vi "pulse_generator_data.vi"(3 "PG Data":refnum<vi>, 4 "Record dP Data":refnum<vi>, 5 "queue in":refnum<queue>, 6 "Stop! Refnum":refnum<vi>, 7 "Recording Progressbar":refnum<vi>, 8 "Seesion Start Time":timestamp, 9 "Pulse Generator Chart Refnums":T3, 10 "Pulse Generator Offsets and Data Saving Controls Refnums":T2, 11 "Pulse Generator Measurement Refnums":T1) -> ()   [LabVIEW 2017]
uses:
  pulse_generator_data_charts_refnums.ctl
  pulse_generator_data_controls_refnums.ctl
  pulse_generator_data_refnums.ctl
  <vilib>/Waveform/WDTOps.llb/WDT Get Waveform Time Array DBL.vi
panel:
  out "size(s)":i32[](graph)
  out "Sampling Rate":refnum<vi>
  out "Recording Duration":refnum<vi>
  out "Camera Voltage Chart":refnum<vi>
  out "Abs Tank Pressure Chart":refnum<vi>
  out "Pitot dP Chart":refnum<vi>
  out "Pulse Generator to Test Section dP Chart":refnum<vi>
  out "W1-7 dP":refnum<vi>
  out "W1-4 dP":refnum<vi>
  out "Mass Flow Rate":refnum<vi>
  out "Liquid Sat Pressure":refnum<vi>
  out "Liquid Temperature":refnum<vi>
  out "Vapor Sat Pressure":refnum<vi>
  out "Vapor Temperature":refnum<vi>
  out "Pitot dP":refnum<vi>
  out "PG to TS dP":refnum<vi>
  out "Pitot Current":refnum<vi>
  out "PG Abs Pressure":refnum<vi>
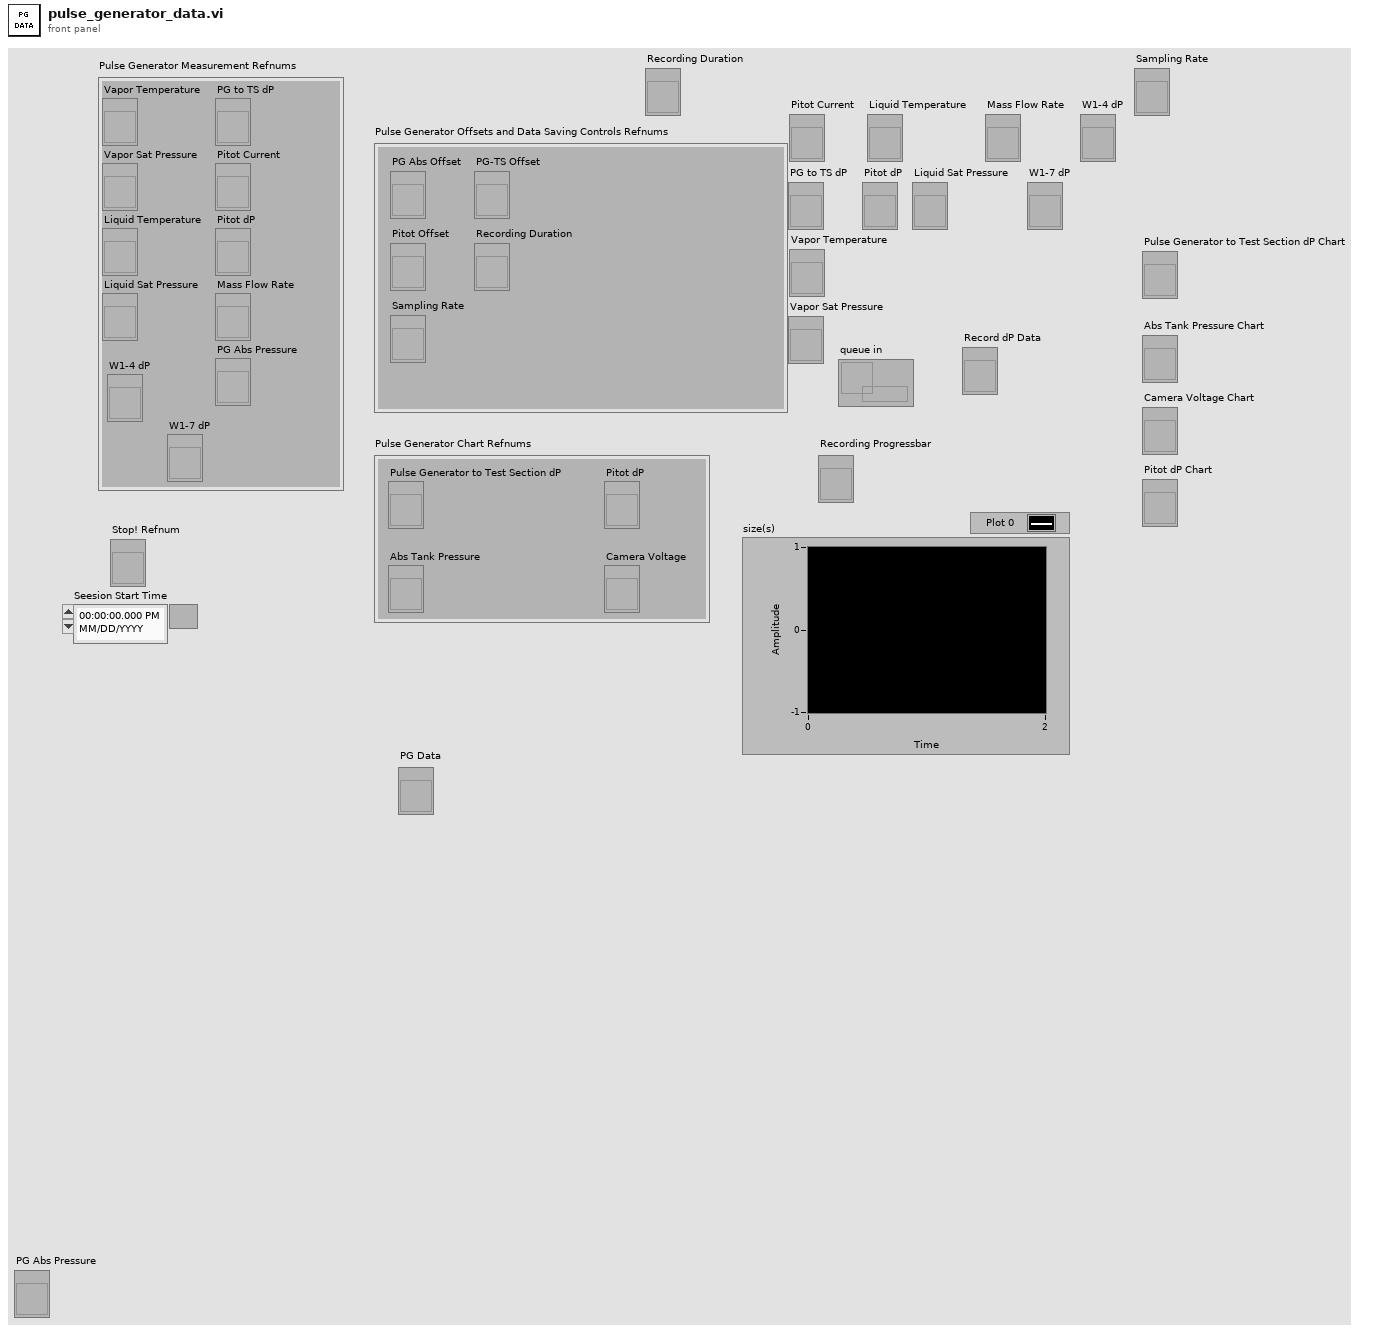
[diagram p1: front panel]
types:
  T1 = typedef "pulse_generator_data_refnums.ctl" = cluster{"Vapor Temperature":refnum<vi>, "Vapor Sat Pressure":refnum<vi>, "Liquid Temperature":refnum<vi>, "Liquid Sat Pressure":refnum<vi>, "PG to TS dP":refnum<vi>, "Pitot Current":refnum<vi>, "Pitot dP":refnum<vi>, "Mass Flow Rate":refnum<vi>, "PG Abs Pressure":refnum<vi>, "W1-4 dP":refnum<vi>, "W1-7 dP":refnum<vi>}
  T2 = typedef "pulse_generator_data_controls_refnums.ctl" = cluster{"PG Abs Offset":refnum<vi>, "Pitot Offset":refnum<vi>, "PG-TS Offset":refnum<vi>, "Recording Duration":refnum<vi>, "Sampling Rate":refnum<vi>}
  T3 = typedef "pulse_generator_data_charts_refnums.ctl" = cluster{"Pulse Generator to Test Section dP":refnum<vi>, "Pitot dP":refnum<vi>, "Abs Tank Pressure":refnum<vi>, "Camera Voltage":refnum<vi>}
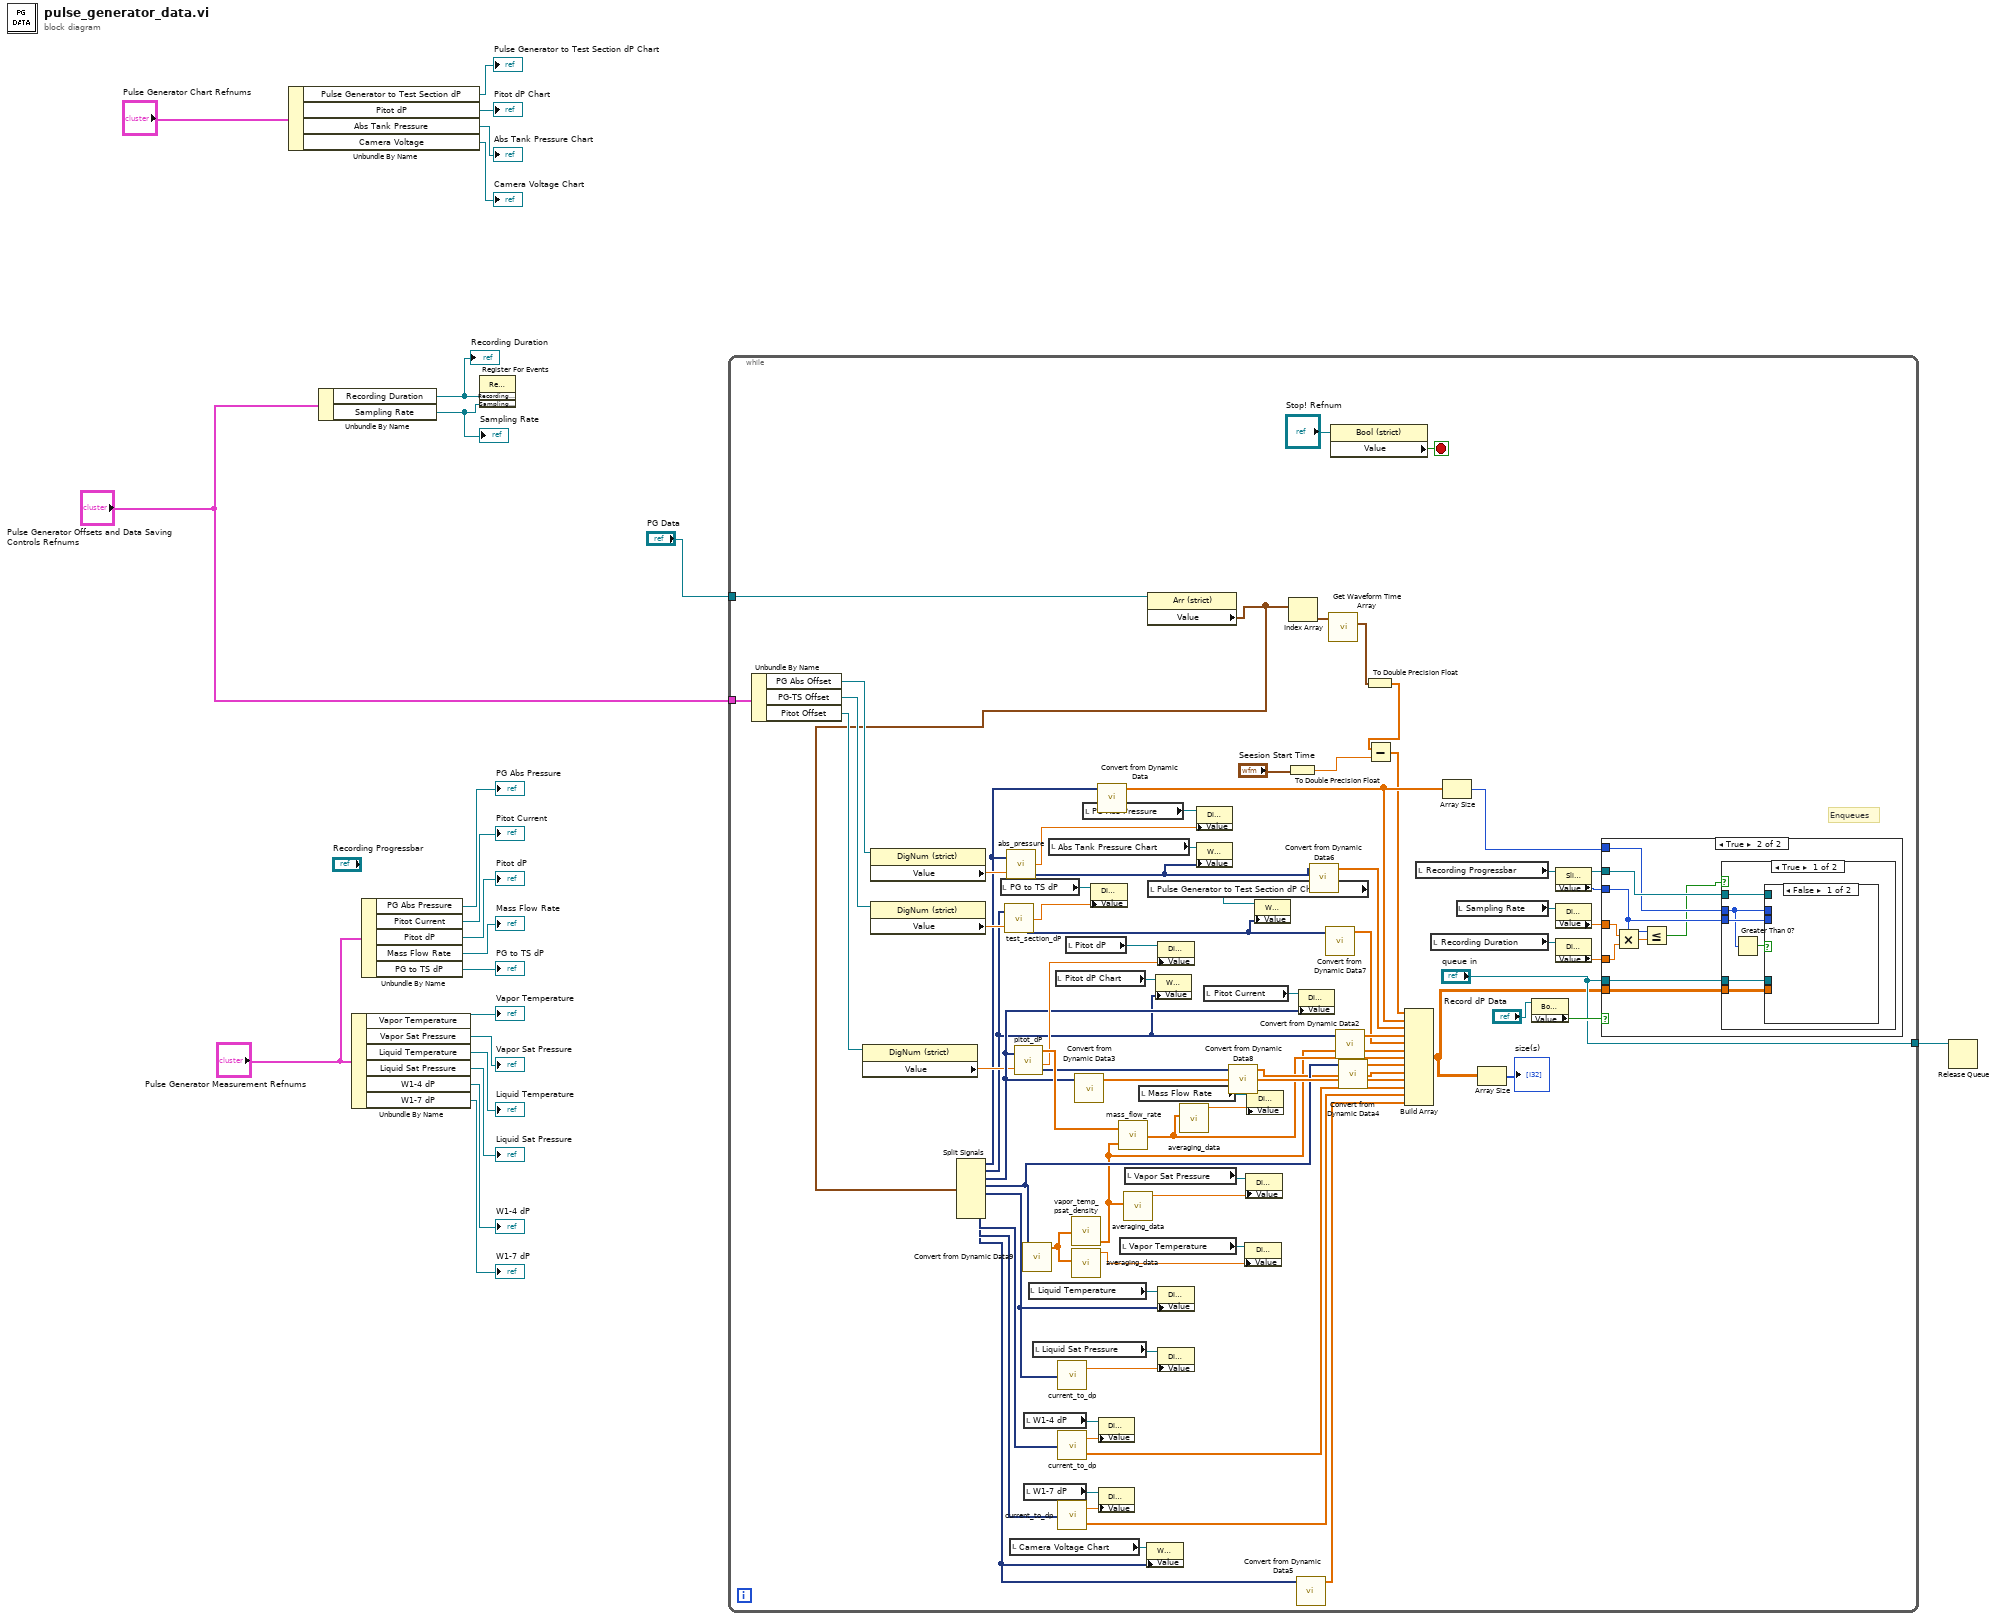
[diagram p0: block diagram]
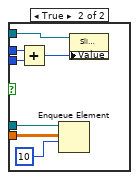
[diagram p3: hidden frame]
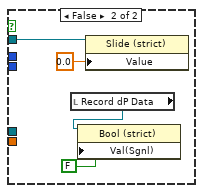
[diagram p4: hidden frame]
diagram:
  n1 = Unbundle By Name("Pulse Generator Chart Refnums") -> ("Pulse Generator to Test Section dP"=→"Pulse Generator to Test Section dP Chart":refnum<vi>, "Pitot dP"=→"Pitot dP Chart":refnum<vi>, "Abs Tank Pressure"=→"Abs Tank Pressure Chart":refnum<vi>, "Camera Voltage"=→"Camera Voltage Chart":refnum<vi>)
  n2 = Unbundle By Name("Pulse Generator Offsets and Data Saving Controls Refnums") -> ("Recording Duration"=w4:refnum<vi>, "Sampling Rate"=w3:refnum<vi>)
  "Recording Duration" <- w4
  "Sampling Rate" <- w3
  n3 = Unbundle By Name("Pulse Generator Measurement Refnums") -> ("Vapor Temperature"=→"Vapor Temperature":refnum<vi>, "Vapor Sat Pressure"=→"Vapor Sat Pressure":refnum<vi>, "Liquid Temperature"=→"Liquid Temperature":refnum<vi>, "Liquid Sat Pressure"=→"Liquid Sat Pressure":refnum<vi>, "W1-4 dP"=→"W1-4 dP":refnum<vi>, "W1-7 dP"=→"W1-7 dP":refnum<vi>)
  n4 = Unbundle By Name("Pulse Generator Measurement Refnums") -> ("PG Abs Pressure"=→"PG Abs Pressure":refnum<vi>, "Pitot Current"=→"Pitot Current":refnum<vi>, "Pitot dP"=→"Pitot dP":refnum<vi>, "Mass Flow Rate"=→"Mass Flow Rate":refnum<vi>, "PG to TS dP"=→"PG to TS dP":refnum<vi>)
  n5 = register-events(w4, w3) -> ()  [unwired: 2 in, 2 out]
  n6 = while {
    tunnel: "Pulse Generator Offsets and Data Saving Controls Refnums" -> [w99]
    tunnel: ["queue in"] -> w6
    tunnel: "PG Data" -> [w30]
    stop <- w100 stop-if-true
    # "Enqueues"
    n7 = Unbundle By Name(w99) -> ("PG Abs Offset"=w98:refnum<vi>, "PG-TS Offset"=w97:refnum<vi>, "Pitot Offset"=w96:refnum<vi>)
    n8 = property class="DigNum (strict)"(reference=w96) -> ("Value"=w48:dbl)  [unwired: 1 in, 2 out]
    n9 = property class="DigNum (strict)"(reference=w98) -> ("Value"=w95:dbl)  [unwired: 1 in, 2 out]
    n10 = property class="DigNum (strict)"(reference=w97) -> ("Value"=w52:dbl)  [unwired: 1 in, 2 out]
    n11 = local read "PG to TS dP"() -> (w94:refnum<vi>)
    n12 = local read "Camera Voltage Chart"() -> (w73:refnum<vi>)
    n13 = local read "W1-4 dP"() -> (w83:refnum<vi>)
    n14 = local read "W1-7 dP"() -> (w80:refnum<vi>)
    n15 = local read "Liquid Temperature"() -> (w87:refnum<vi>)
    n16 = local read "Liquid Sat Pressure"() -> (w89:refnum<vi>)
    n17 = local read "Abs Tank Pressure Chart"() -> (w76:refnum<vi>)
    n18 = local read "Pitot dP Chart"() -> (w75:refnum<vi>)
    n19 = local read "Pitot dP"() -> (w92:refnum<vi>)
    n20 = local read "PG Abs Pressure"() -> (w50:refnum<vi>)
    n21 = local read "Vapor Temperature"() -> (w85:refnum<vi>)
    n22 = local read "Vapor Sat Pressure"() -> (w78:refnum<vi>)
    n23 = local read "Mass Flow Rate"() -> (w90:refnum<vi>)
    n24 = property class="Arr (strict)"(reference=w30) -> ("Value"=w29:waveform(dbl)[])  [unwired: 1 in, 2 out]
    n25 = Split Signals(w29) -> (w37:dynamicdata, w46:dynamicdata, w55:dynamicdata, w53:dynamicdata, w86:dynamicdata, w82:dynamicdata, w81:dynamicdata, w64:dynamicdata)  [unwired: 8 in]
    n26 = call "test_section_dP.vi"("dP Voltage"=w46, "Offset[Pa]"=w52) -> ("Adj dP"=w71:dbl, "Adj dP Array"=w40:dynamicdata)  [unwired: 1 out]
    n27 = call "abs_pressure.vi"("Input Voltage"=w37, "Offset[Pa]"=w95) -> ("Adj Absolute Pressure"=w72:dbl, "Adj Absolute Pressure Array"=w42:dynamicdata)  [unwired: 1 out]
    n28 = call "pitot_dP.vi"("Pitot Current"=w55, "Pitot Offset [Pa]"=w48) -> ("dP H2O"=w91:dbl[], "Adj dP [Pa]"=w74:dbl, "Adj dP [Pa] Array"=w38:dynamicdata)  [unwired: 1 out]
    n29 = call "Convert from Dynamic Data9"("Dynamic Data Type"=w53) -> ("Array"=w26:dbl[])  [unwired: 3 in]
    n30 = call "current_to_dp.vi"("Current [A]"=w86) -> ("dP [Pa]"=w88:dbl)  [unwired: 1 out]
    n31 = call "current_to_dp.vi"("Current [A]"=w82) -> ("dP [Pa]"=w84:dbl, "dP Array [Pa]"=w70:dbl[])
    n32 = call "current_to_dp.vi"("Current [A]"=w81) -> ("dP [Pa]"=w79:dbl, "dP Array [Pa]"=w54:dbl[])
    n33 = call "vapor_temp_psat_density.vi"("Vapor Temp [C]"=w26) -> ("Vapor Density"=w24:dbl[])  [unwired: 1 in, 1 out]
    n34 = call "averaging_data.vi"("Input"=w26) -> ("Average"=w25:dbl)  [unwired: 6 in, 3 out]
    n35 = call "Convert from Dynamic Data3"("Dynamic Data Type"=w55) -> ("Array"=w67:dbl[])  [unwired: 3 in]
    n36 = property class="DigNum (strict)"(reference=w94, "Value"=w71) -> ()  [unwired: 1 in, 2 out]
    n37 = call "Convert from Dynamic Data"("Dynamic Data Type"=w37) -> ("Array"=w63:dbl[])  [unwired: 3 in]
    n38 = property class="DigNum (strict)"(reference=w83, "Value"=w84) -> ()  [unwired: 1 in, 2 out]
    n39 = property class="DigNum (strict)"(reference=w80, "Value"=w79) -> ()  [unwired: 1 in, 2 out]
    n40 = call "mass_flow_rate.vi"("Density"=w24, "dP Pa"=w91) -> ("Mass Flow Rate [g/s] Array"=w27:dbl[])
    n41 = call "averaging_data.vi"("Input"=w24) -> ("Average"=w23:dbl)  [unwired: 6 in, 3 out]
    n42 = property class="WFChart (strict)"(reference=w73, "Value"=w64) -> ()  [unwired: 1 in, 2 out]
    n43 = local read "Pulse Generator to Test Section dP Chart"() -> (w77:refnum<vi>)
    n44 = property class="WFChart (strict)"(reference=w75, "Value"=w46) -> ()  [unwired: 1 in, 2 out]
    n45 = property class="DigNum (strict)"(reference=w92, "Value"=w74) -> ()  [unwired: 1 in, 2 out]
    n46 = property class="DigNum (strict)"(reference=w87, "Value"=w86) -> ()  [unwired: 1 in, 2 out]
    n47 = property class="DigNum (strict)"(reference=w89, "Value"=w88) -> ()  [unwired: 1 in, 2 out]
    n48 = call "averaging_data.vi"("Input"=w27) -> ("Average"=w28:dbl)  [unwired: 6 in, 3 out]
    n49 = property class="DigNum (strict)"(reference=w50, "Value"=w72) -> ()  [unwired: 1 in, 2 out]
    n50 = property class="WFChart (strict)"(reference=w76, "Value"=w42) -> ()  [unwired: 1 in, 2 out]
    n51 = local read "Pitot Current"() -> (w93:refnum<vi>)
    n52 = call "Convert from Dynamic Data8"("Dynamic Data Type"=w38) -> ("Array"=w39:dbl[])  [unwired: 3 in]
    n53 = property class="DigNum (strict)"(reference=w85, "Value"=w25) -> ()  [unwired: 1 in, 2 out]
    n54 = property class="DigNum (strict)"(reference=w78, "Value"=w23) -> ()  [unwired: 1 in, 2 out]
    n55 = property class="DigNum (strict)"(reference=w90, "Value"=w28) -> ()  [unwired: 1 in, 2 out]
    n56 = property class="WFChart (strict)"(reference=w77, "Value"=w40) -> ()  [unwired: 1 in, 2 out]
    n57 = To Double Precision Float(number="Seesion Start Time") -> (double precision float=w32:dbl)
    n58 = Index Array(array=w29) -> (element=w36:waveform(dbl))  [unwired: 1 in]
    n59 = call "Convert from Dynamic Data5"("Dynamic Data Type"=w64) -> ("Array"=w65:dbl[])  [unwired: 3 in]
    n60 = property class="DigNum (strict)"(reference=w93, "Value"=w55) -> ()  [unwired: 1 in, 2 out]
    n61 = call "Convert from Dynamic Data6"("Dynamic Data Type"=w42) -> ("Array"=w43:dbl[])  [unwired: 3 in]
    n62 = call "Convert from Dynamic Data7"("Dynamic Data Type"=w40) -> ("Array"=w41:dbl[])  [unwired: 3 in]
    n63 = call-poly <vilib>:"Get Waveform Time Array.vi"("waveform in"=w36) -> ("X array"=w35:timestamp[])  [unwired: 9 in, 1 out]
    n64 = property class="Bool (strict)"(reference="Stop! Refnum") -> ("Value"=w100:bool)  [unwired: 1 in, 2 out]
    n65 = call "Convert from Dynamic Data2"("Dynamic Data Type"=w46) -> ("Array"=w68:dbl[])  [unwired: 3 in]
    n66 = call "Convert from Dynamic Data4"("Dynamic Data Type"=w53) -> ("Array"=w66:dbl[])  [unwired: 3 in]
    n67 = To Double Precision Float(number=w35) -> (double precision float=w34:dbl[])
    n68 = Subtract(x=w34, y=w32) -> (x-y=w31:dbl[])
    n69 = Build Array(w31, w63, w43, w68, w41, w24, w27, w66, w39, w67, w70, w54, w65) -> (w45:dbl[][])
    n70 = local read "Recording Progressbar"() -> (w57:refnum<vi>)
    n71 = local read "Recording Duration"() -> (w61:refnum<vi>)
    n72 = Array Size(array=w63) -> (size(s)=w49:i32)
    n73 = local read "Sampling Rate"() -> (w62:refnum<vi>)
    n74 = Array Size(array=w45) -> (size(s)=→"size(s)":i32[])
    n75 = property class="Bool (strict)"(reference="Record dP Data") -> ("Value"=w51:bool)  [unwired: 1 in, 2 out]
    n76 = property class="Slide (strict)"(reference=w57) -> (reference out=w56:refnum<vi>, "Value"=w58:u32)  [unwired: 1 in, 1 out]
    n77 = property class="DigNum (strict)"(reference=w62) -> ("Value"=w60:dbl)  [unwired: 1 in, 2 out]
    n78 = property class="DigNum (strict)"(reference=w61) -> ("Value"=w59:dbl)  [unwired: 1 in, 2 out]
    n79 = case shown="True" w51 {
      tunnel: "queue in" -> [_ w110]
      tunnel: w49 -> [_ w103]
      tunnel: w60 -> [_ w109]
      tunnel: w59 -> [_ w108]
      tunnel: w58 -> [_ w106]
      tunnel: w56 -> [_ w105]
      tunnel: w45 -> [_ w104]
      frame False {
      }
      frame True {
        n80 = Multiply(x=w109, y=w108) -> (x*y=w107:dbl)
        n81 = Less Or Equal?(x=w106, y=w107) -> (x <= y?=w102:bool)
        n82 = case shown="True" w102 {
          tunnel: w110 -> [w116 _]
          tunnel: w105 -> [w115 w127]
          tunnel: w106 -> [w114 _]
          tunnel: w103 -> [w111 _]
          tunnel: w104 -> [w113 _]
          frame True {
            n83 = Greater Than 0?(x=w111) -> (x > 0?=w112:bool)
            n84 = case shown="False" w112 {
              tunnel: w116 -> [_ w122]
              tunnel: w115 -> [_ w121]
              tunnel: w114 -> [_ w119]
              tunnel: w111 -> [_ w118]
              tunnel: w113 -> [_ w117]
              frame False {
              }
              frame True {
                n85 = Add(x=w118, y=w119) -> (x+y=w120:u32)
                n86 = Enqueue Element(queue=w122, element=w117, timeout in ms (-1)=10) -> ()  [unwired: 1 in, 3 out]
                n87 = property class="Slide (strict)"(reference=w121, "Value"=w120) -> ()  [unwired: 1 in, 2 out]
              }
            }
          }
          frame False {
            n88 = local read "Record dP Data"() -> (w124:refnum<vi>)
            n89 = property class="Bool (strict)"(reference=w124, "Val(Sgnl)"=FALSE ("Value (Signaling)")) -> ()  [unwired: 1 in, 2 out]
            n90 = property class="Slide (strict)"(reference=w127, "Value"=0.0) -> ()  [unwired: 1 in, 2 out]
          }
        }
      }
    }
  }
  n91 = Release Queue(queue=w6) -> ()  [unwired: 2 in, 3 out]
